vi "Ball Intake System.vi"(0 "Ball System Actions":T1) -> ()   [LabVIEW 2019]
uses:
  Controls/Ball System Actions.ctl
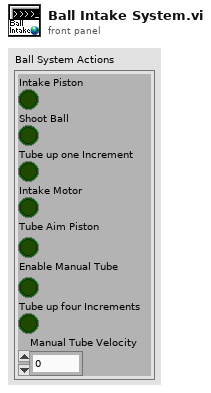
[diagram p1: front panel]
types:
  T1 = typedef "Ball System Actions.ctl" = cluster{"Intake Piston ":bool, "Shoot Ball":bool, "Tube up one Increment\t":bool, "Intake Motor\t":bool, "Tube Aim Piston":bool, "Enable Manual Tube":bool, "Tube up four Increments":bool, "Manual Tube Velocity":dbl}
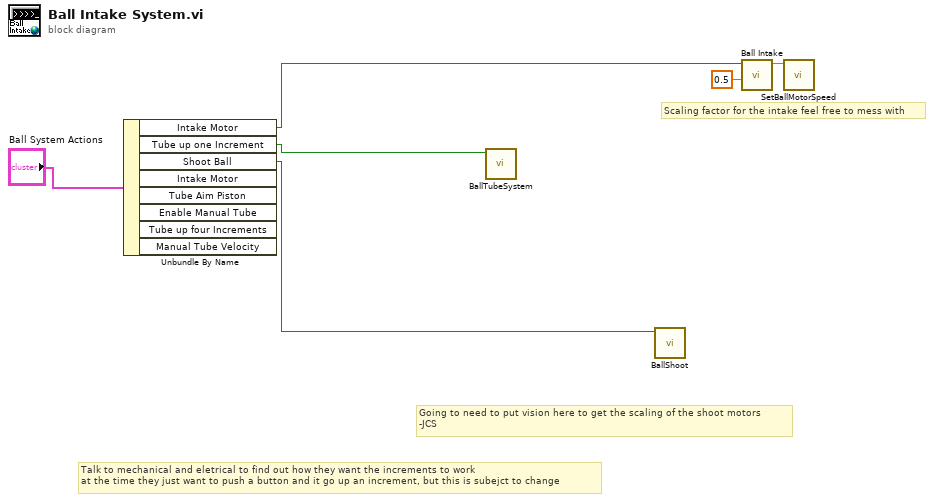
[diagram p0: block diagram]
diagram:
  # "Scaling factor for the intake feel free to mess with"
  # "Talk to mechanical and eletrical to find out how they want the increments to work\nat the time they just want to push a button and it go up an increment, but this is subejct to change"
  # "Going to need to put vision here to get the scaling of the shoot motors\n-JCS"
  n1 = Unbundle By Name("Ball System Actions") -> ("Intake Motor"=w3:bool, "Tube up one Increment"=w2:bool, "Shoot Ball"=w4:bool)  [unwired: 5 out]
  n2 = call "BallTubeSystem.vi"("Tube up one Increment"=w2) -> ()  [unwired: 9 in, 1 out]
  n3 = call "BallShoot.vi"("Shoot ball"=w4) -> ()  [unwired: 11 in]
  n4 = call "Ball Intake.vi"("Scaling factor"=0.5, "Intake"=w3) -> ("IntakeSpeed"=w6:dbl)  [unwired: 9 in]
  n5 = call "SetBallMotorSpeed.vi"("IntakeSpeed"=w6) -> ()  [unwired: 11 in]
